vi "PRIME FITS Offsets.vi"(8 "error in (no error)":errorcluster, 10 "Offsets":u16[](array[numeric]) format="%.0x", 11 "gfits refnum":T1) -> (0 "error out":errorcluster, 3 "gfits refnum out":T1)   [LabVIEW 2021, in "PRIME Detector.lvclass"]
uses:
  PRIME Detector.lvclass
  <userlib>/gfitsio/gfitsio-refnum.ctl
  <userlib>/gfitsio/gfitsio-write-key-string.vi
  PRIME Detector.lvclass/PRIME Detector.ctl
  <userlib>/gfitsio/gfitsio.lvlib
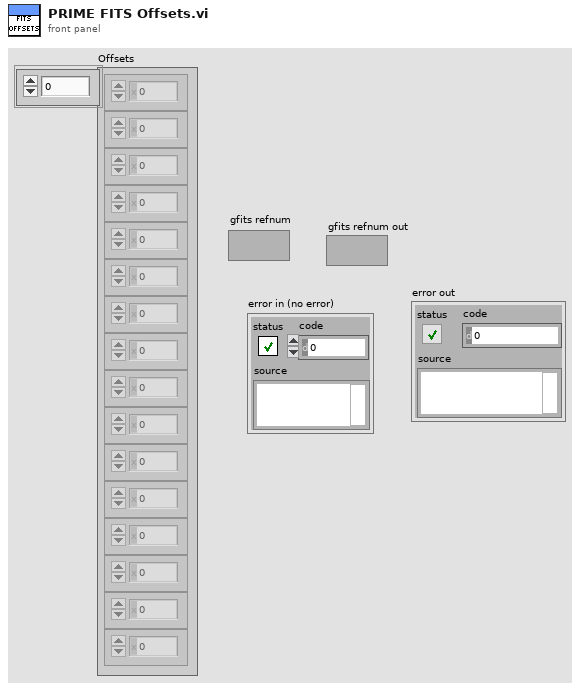
[diagram p1: front panel]
types:
  T1 = typedef "gfitsio.lvlib/gfitsio-refnum.ctl" = refnum<k1>
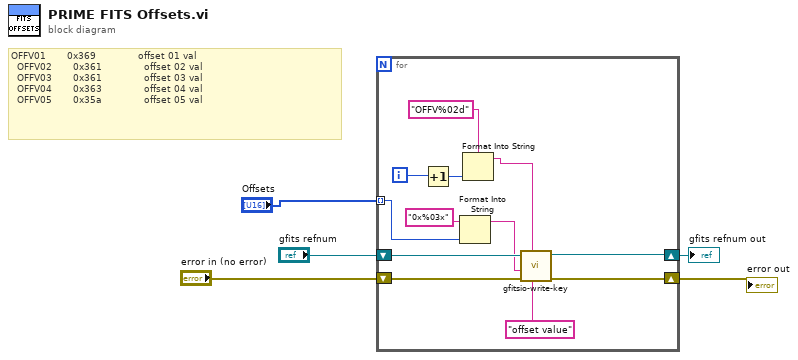
[diagram p0: block diagram]
diagram:
  # "OFFV01       0x369              offset 01 val\n  OFFV02       0x361              offset 02 val\n  OFFV03       0x361              offset 03 val\n  OFFV04       0x363              offset 04 val\n  OFFV05       0x35a              offset 05 val"
  n1 = for {
    tunnel: "Offsets" -> [w9] mode=indexing
    shift-right: [w13] -> w3
    shift-left: "gfits refnum" -> [w14]
    shift-right: [w6] -> w1
    shift-left: "error in (no error)" -> [w7]
    i -> [w16]
    n2 = Increment(x=w16) -> (x+1=w15:i32)
    n3 = Format Into String(initial string="0x%03x" ("format string"), w9) -> (resulting string=w8:string)  [unwired: 2 in, 1 out]
    n4 = Format Into String(format string="OFFV%02d", w15) -> (resulting string=w11:string)  [unwired: 2 in, 1 out]
    n5 = call-poly <userlib>:"gfitsio-write-key.vi"("comment"="offset value", "keyname"=w11, "error in (no error)"=w7, "value"=w8, "gfits refnum"=w14) -> ("error out"=w6:errorcluster, "dup gfits refnum"=w13:T1)  [unwired: 5 in]
  }
  "gfits refnum out" <- w3
  "error out" <- w1
